vi "Overlord_test.vi"() -> ()   [LabVIEW 2014]
panel:
  in  "Arduino_IP":string
  out "Transport_Motor":string
  out "Transport":string
  out "Winch PW":string
  out "Drum PW":string
  out "Scoop PW":string
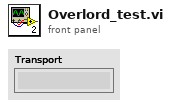
[diagram p1: front panel]
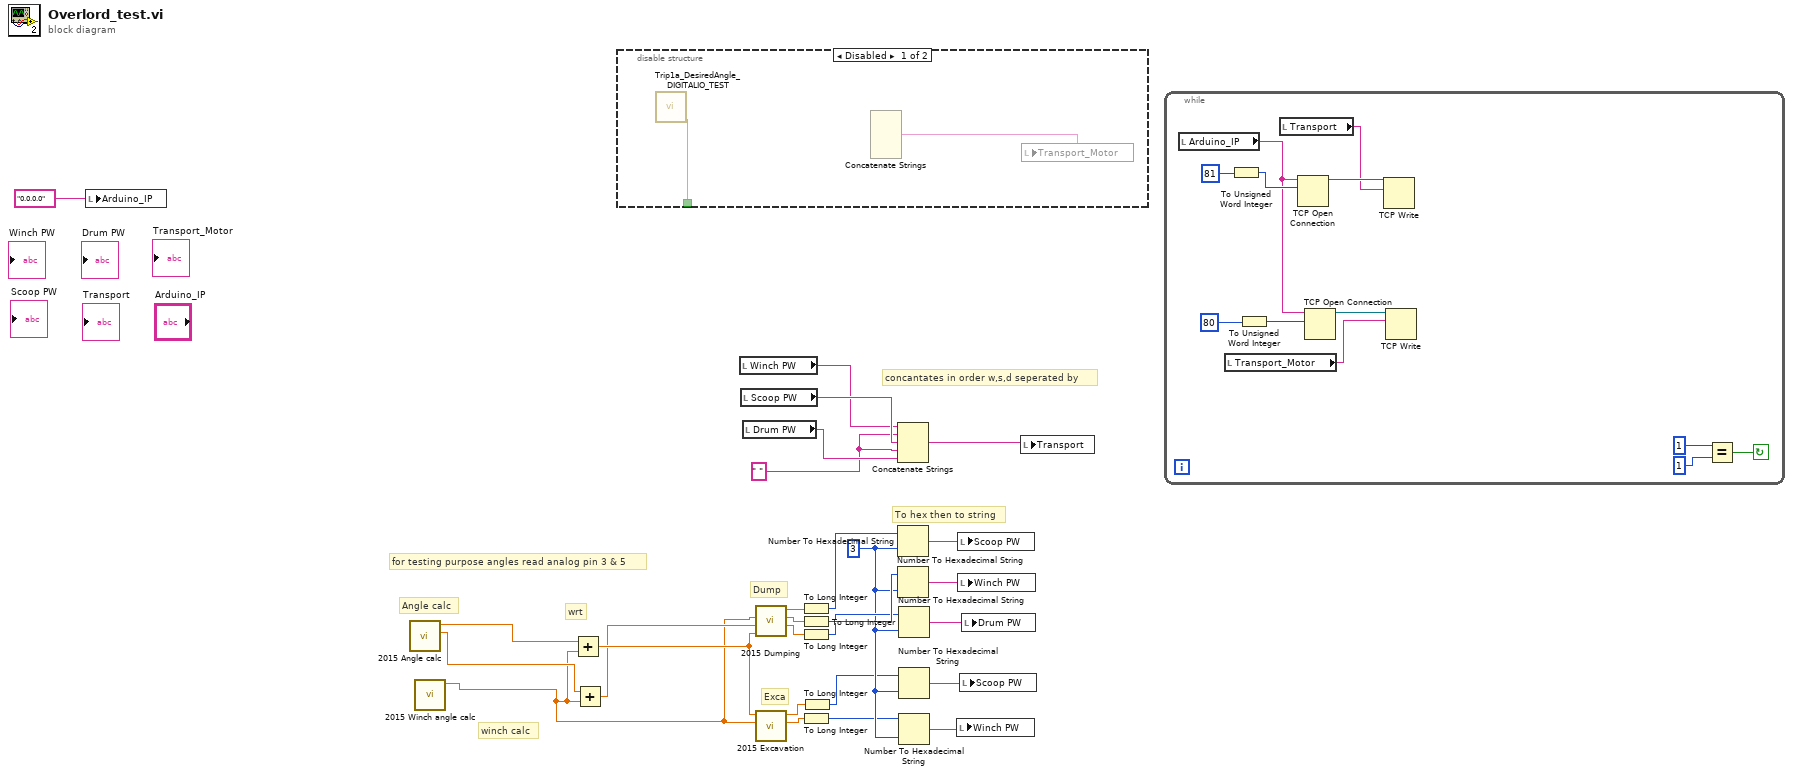
[diagram p0: block diagram]
diagram:
  w1 = " "
  w17 = 3
  # "To hex then to string"
  # "concantates in order w,s,d seperated by"
  # "winch calc"
  # "wrt"
  # "Exca"
  # "Dump"
  # "for testing purpose angles read analog pin 3 & 5"
  # "Angle calc"
  n1 = local write "Arduino_IP"("0.0.0.0") -> ()
  n2 = call "2015 Angle calc.vi"() -> ("Drum angle"=w27:dbl, "Scoop angle"=w26:dbl)  [unwired: 10 in]
  n3 = call "2015 Winch angle calc.vi"() -> ("Winch angle"=w5:dbl)  [unwired: 11 in]
  n4 = Add(x=w26, y=w5) -> (x+y=w25:dbl)
  n5 = Add(x=w27, y=w5) -> (x+y=w24:dbl)
  n6 = disable-structure shown="Disabled" {
    disable-tunnel: [w28 _] -> _
    frame Disabled {
      n7 = call "Trip1a_DesiredAngle_DIGITALIO_TEST.vi"() -> ("Commence Mining"=w28:bool)  [unwired: 11 in]
      n8 = Concatenate Strings() -> (w29:string)  [unwired: 6 in]
      n9 = local write "Transport_Motor"(w29) -> ()
    }
    frame Enabled {
    }
  }
  n10 = local read "Winch PW"() -> (w2:string)
  n11 = local read "Scoop PW"() -> (w3:string)
  n12 = local read "Drum PW"() -> (w4:string)
  n13 = call "2015 Dumping.vi"("Scoop angle"=w25, "Drum angle"=w24, "Winch angle"=w5) -> ("Drum PW"=w20:dbl, "Winch PW"=w21:dbl, "Scoop PW"=w23:dbl)  [unwired: 4 in, 1 out]
  n14 = call "2015 Excavation.vi"("Winch angle"=w5, "Scoop angle"=w25) -> ("Winch PW"=w15:dbl, "Scoop PW"=w16:dbl)  [unwired: 8 in]
  n15 = To Long Integer(number=w23) -> (32bit integer=w22:i32)
  n16 = To Long Integer(number=w21) -> (32bit integer=w19:i32)
  n17 = To Long Integer(number=w20) -> (32bit integer=w18:i32)
  n18 = To Long Integer(number=w15) -> (32bit integer=w13:i32)
  n19 = To Long Integer(number=w16) -> (32bit integer=w14:i32)
  n20 = Concatenate Strings(w2, w1, w3, w1, w4) -> (w7:string)
  n21 = Number To Hexadecimal String(1:w17, 2:w22) -> (0:w12:string)
  n22 = Number To Hexadecimal String(1:w17, 2:w19) -> (0:w11:string)
  n23 = Number To Hexadecimal String(1:w17, 2:w18) -> (0:w10:string)
  n24 = Number To Hexadecimal String(1:w17, 2:w14) -> (0:w9:string)
  n25 = Number To Hexadecimal String(1:w17, 2:w13) -> (0:w8:string)
  n26 = local write "Winch PW"(w8) -> ()
  n27 = local write "Scoop PW"(w12) -> ()
  n28 = local write "Winch PW"(w11) -> ()
  n29 = local write "Scoop PW"(w9) -> ()
  n30 = local write "Drum PW"(w10) -> ()
  n31 = local write "Transport"(w7) -> ()
  n32 = while {
    stop <- w37 continue-if-true
    n33 = local read "Arduino_IP"() -> (w33:string)
    n34 = local read "Transport_Motor"() -> (w30:string)
    n35 = To Unsigned Word Integer(number=81) -> (unsigned 16bit integer=w40:u16)
    n36 = To Unsigned Word Integer(number=80) -> (unsigned 16bit integer=w31:u16)
    n37 = local read "Transport"() -> (w38:string)
    n38 = TCP Open Connection(address=w33, remote port or service name=w40) -> (connection ID=w39:refnum<k5>)  [unwired: 3 in, 1 out]
    n39 = TCP Open Connection(address=w33, remote port or service name=w31) -> (connection ID=w34:refnum<k5>)  [unwired: 3 in, 1 out]
    n40 = TCP Write(connection ID=w39, data in=w38) -> ()  [unwired: 2 in, 3 out]
    n41 = TCP Write(connection ID=w34, data in=w30) -> ()  [unwired: 2 in, 3 out]
    n42 = Equal?(x=1, y=1) -> (x = y?=w37:bool)
  }
